vi "FTW-Message-Request-Reply.vi"(8 "error in":errorcluster, 11 "FTW Incoming Request":refnum<class "FTW-Message-IncomingRequest.lvclass">) -> (0 "error out":errorcluster, 2 "Timed out?":bool)   [LabVIEW 2013, in "FTW-Message-IncomingRequest.lvclass"]
uses:
  FTW-Message-IncomingRequest.lvclass
  FTW-Message-IncomingRequest.lvclass/FTW-Message-IncomingRequest.ctl
  Endpoint/FTW-Endpoint.lvclass
panel:
  # "Inputs"
  # "Outputs"
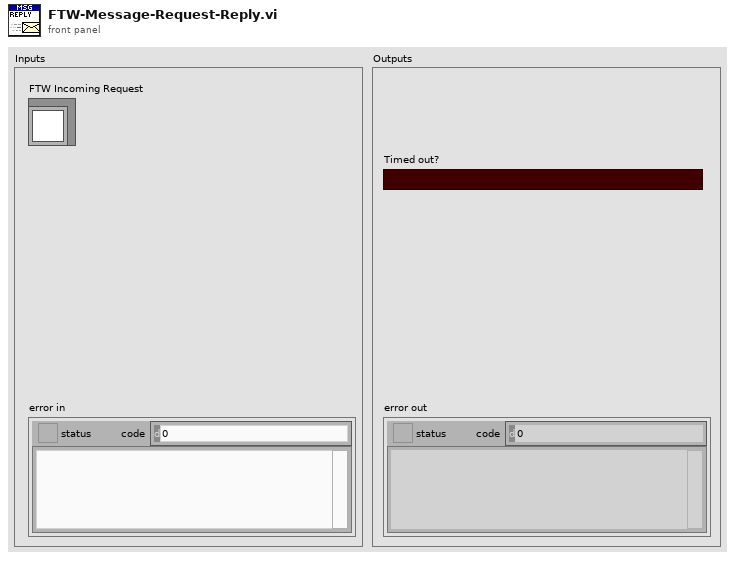
[diagram p1: front panel]
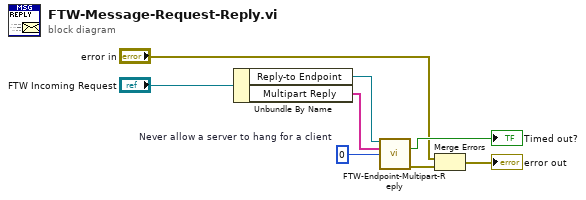
[diagram p0: block diagram]
diagram:
  w5 = 0  # Never allow a server to hang for a client
  n1 = Unbundle By Name("FTW Incoming Request") -> ("Reply-to Endpoint"=w7:refnum<class "FTW-Endpoint.lvclass">, "Multipart Reply"=w3:string[])
  n2 = call-dynamic "FTW-Endpoint-Multipart-Reply.vi"("FTW Endpoint"=w7, "Multipart Message"=w3, "Timeout"=w5) -> ("Timed out?"=→"Timed out?":bool, "error out"=w6:errorcluster)  [unwired: 10 in, 1 out]
  n3 = Merge Errors("error in", w6) -> (→"error out":errorcluster)
